vi "GetDeviceTypeConfigSection.vi"(9 "key":string, 10 "key values":T2[](array[typedef])) -> (2 "key value pairs out":T1[](array[typedef]), 5 "found":bool)   [LabVIEW 2017, in "PropertyHelpers.lvlib"]
doc: "Returns the name-value pairs of properties defined for a particular process in a software configuration. Use this VI to get the properties returned by the Get Device Type Configuration VI."
uses:
  <vilib>/addons/InsightCM/Utilities/PropertyHelpers/PropertyHelpers.lvlib
  <vilib>/addons/InsightCM/MessageBus/Base/controls/SectionKeyValues.ctl
  <vilib>/addons/InsightCM/MessageBus/Base/controls/KeyValuePair.ctl
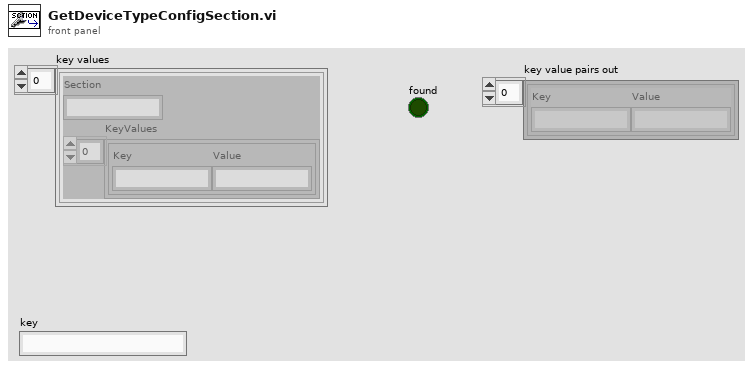
[diagram p1: front panel]
types:
  T1 = typedef "KeyValuePair.ctl" = cluster{"Key":string, "Value":string}
  T2 = typedef "SectionKeyValues.ctl" = cluster{"Section":string, "KeyValues":T1[]}
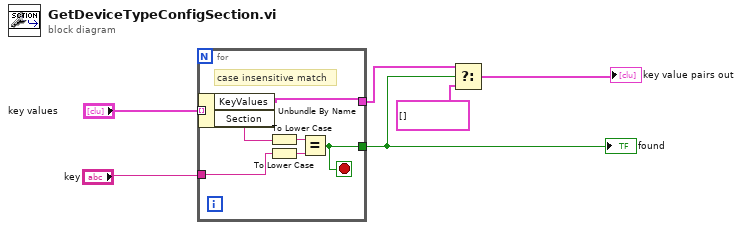
[diagram p0: block diagram]
diagram:
  n1 = for {
    tunnel: "key values" -> [w13] mode=indexing
    tunnel: "key" -> [w8]
    tunnel: [w12] -> w2
    tunnel: [w7] -> w6
    stop <- w12 stop-if-true
    # "case insensitive match"
    n2 = Unbundle By Name(w13) -> ("KeyValues"=w7:T1[], "Section"=w11:string)
    n3 = To Lower Case(string=w11) -> (all lower case string=w10:string)
    n4 = To Lower Case(string=w8) -> (all lower case string=w9:string)
    n5 = Equal?(x=w10, y=w9) -> (x = y?=w12:bool)
  }
  "found" <- w2
  n6 = Select(t=w6, s=w2, f=T1[] [] ("key value pairs out")) -> (s? t:f=→"key value pairs out":T1[])
